vi "DriveModuleControl_TravTuneKsKv.vi"(8 "error in":errorcluster, 9 "Actual State":T1={"Speed"=0.0, "Angle"={"VALUE"=0.0, "COS"=1.0, "SIN"=0.0}} {"Angle"."SIN" format="%13.4f"; "Angle"."COS" format="%13.4f"; "Angle"."VALUE" format="%13.4f"}, 10 "Desired State":T1={"Speed"=0.0, "Angle"={"VALUE"=0.0, "COS"=1.0, "SIN"=0.0}} {"Angle"."SIN" format="%13.4f"; "Angle"."COS" format="%13.4f"; "Angle"."VALUE" format="%13.4f"}, 11 "ModualNamePrefix":i32) -> (0 "error out":errorcluster)   [LabVIEW 2023]
uses:
  <vilib>/Rock Robotics/WPI/ThirdParty/JAS_Junk/TrajLib/TypeDef/SWERVE_DRIVE_MODULE_STATE.ctl
  <vilib>/Rock Robotics/WPI/ThirdParty/JAS_Junk/TrajLib/TypeDef/ROTATION2D.ctl
  <vilib>/Rock Robotics/WPI/ThirdParty/JAS_Junk/TrajLib/LinearFilter_MovingAvg_Execute.vi
  <vilib>/Rock Robotics/WPI/ThirdParty/JAS_Junk/TrajLib/Rotation2d_Minus.vi
  <vilib>/Rock Robotics/WPI/ThirdParty/JAS_Junk/TrajLib/Rotation2d_GetRadians.vi
  <vilib>/Rock Robotics/WPI/ThirdParty/JAS_Junk/TrajLib/SwerveModuleState_New.vi
  <vilib>/Rock Robotics/WPI/ThirdParty/JAS_Junk/TrajLib/Rotation2d_RotateBy.vi
  <vilib>/Rock Robotics/WPI/ThirdParty/JAS_Junk/TrajLib/Rotation2d_CreateAngle.vi
  <vilib>/Rock Robotics/WPI/ThirdParty/JAS_Junk/TrajLib/SimpleMotorFF_Calculate.vi
  <vilib>/Rock Robotics/WPI/ThirdParty/JAS_Junk/TrajLib/LinearFilter_ResetToValue.vi
  <vilib>/Rock Robotics/WPI/ThirdParty/JAS_Junk/TrajLib/LinearFilter_Calculate.vi
  <vilib>/Rock Robotics/WPI/ThirdParty/JAS_Junk/TrajLib/PIDController_AtSetpoint.vi
  <vilib>/Rock Robotics/WPI/ThirdParty/JAS_Junk/TrajLib/PIDController_SetPIDF.vi
  <vilib>/Rock Robotics/WPI/ThirdParty/JAS_Junk/TrajLib/PIDController_SetDerivativeFilter.vi
  <vilib>/Rock Robotics/WPI/ThirdParty/JAS_Junk/TrajLib/PIDController_SetIntegratorRange.vi
  <vilib>/Rock Robotics/WPI/ThirdParty/JAS_Junk/TrajLib/PIDController_SetTolerancePandV.vi
  <vilib>/Rock Robotics/WPI/ThirdParty/JAS_Junk/TrajLib/PIDController_DisableContinousInput.vi
  <vilib>/Rock Robotics/WPI/ThirdParty/JAS_Junk/TrajLib/PIDController_EnableContinousInput.vi
  <vilib>/Rock Robotics/WPI/ThirdParty/JAS_Junk/TrajLib/PIDController_Reset.vi
  <vilib>/Rock Robotics/WPI/ThirdParty/JAS_Junk/TrajLib/PIDController_New.vi
  <vilib>/Rock Robotics/WPI/ThirdParty/JAS_Junk/TrajLib/PIDController_SetOutputLimits.vi
  <vilib>/Rock Robotics/WPI/ThirdParty/JAS_Junk/TrajLib/VI/PIDController_SetIntegratorZone.vi
  <vilib>/Rock Robotics/WPI/ThirdParty/JAS_Junk/TrajLib/Rotation2d_UnaryMinus.vi
  <vilib>/Rock Robotics/WPI/ThirdParty/JAS_Junk/TrajLib/Rotation2d_CreateXY.vi
  <vilib>/Rock Robotics/WPI/ThirdParty/JAS_Junk/TrajLib/PIDController_NewPeriod.vi
  <vilib>/Rock Robotics/WPI/ThirdParty/JAS_Junk/TrajLib/Util_CalcDist.vi
  <vilib>/Rock Robotics/SystemInterfaces/NetworkCommunication/NetComm_UsageReport_report.vi
  <vilib>/Rock Robotics/WPI/ThirdParty/Phoenix6/Phoenix6_Device_RefNumRegistryGet.vi
  <vilib>/Rock Robotics/WPI/MotorControl/WPI_MotorControlRefNum Registry Get.vi
  <vilib>/Rock Robotics/Network Tables/NT Write Number.vi
  DriveGlobal.vi
  <vilib>/Rock Robotics/WPI/ThirdParty/JAS_Junk/TrajLib/Globals/Util_LibraryGlobals.vi
  <vilib>/Rock Robotics/WPI/ThirdParty/JAS_Junk/TrajLib/PIDController_AdvCalculate_FF_Sp_Pv.vi
  <vilib>/Rock Robotics/WPI/ThirdParty/JAS_Junk/TrajLib/LinearFilter_MovingAverage.vi
  <vilib>/Utility/semaphor.llb/Obtain Semaphore Reference.vi
  <vilib>/Rock Robotics/WPI/ThirdParty/JAS_Junk/TrajLib/Timer_Reset.vi
  DriveTuningGlobals.vi
  <vilib>/Rock Robotics/WPI/ThirdParty/JAS_Junk/TrajLib/Trajectory_Library.lvlib
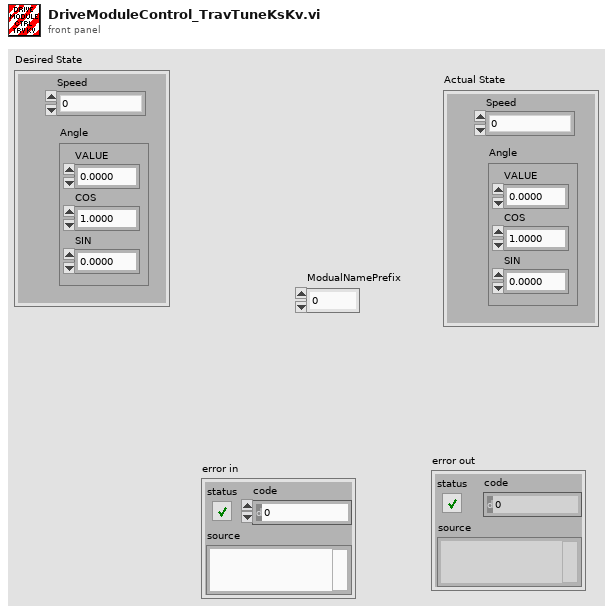
[diagram p1: front panel]
types:
  T1 = typedef "Trajectory_Library.lvlib/SWERVE_DRIVE_MODULE_STATE.ctl" = cluster{"Speed":dbl, "Angle":T2}
  T2 = typedef "Trajectory_Library.lvlib/ROTATION2D.ctl" = cluster{"VALUE":dbl, "COS":dbl, "SIN":dbl}
  T3 = typedef "WPI_MotorControlDeviceRef.ctl" = cluster{"DeviceStatus":errorcluster, "Type":T4, "PWM":cluster{"PWM Channel":T5, "DeadBand":T6}, "CAN":cluster{"Device Number":u8, "SetOutput VI Ref":variant, "GetOutput VI Ref":variant, "Enable VI Ref":variant, "Disable VI Ref":variant, "Data":variant}, "Invert":bool, "DIO PWM":cluster{"PWM \"Enable\" Channel":T5, "DIOChannel":T7, "PWM Rate":dbl}}
  T4 = typedef "WPI_MotorControlType.ctl" = enum16{"PWM", "CAN", "DIO PWM"}
  T5 = typedef "FPGA_DIOPWMChannel.ctl" = enum8{"PWM 0", "PWM 1", "PWM 2", "PWM 3", "PWM 4", "PWM 5", "PWM 6", "PWM 7", "PWM 8", "PWM 9", "PWM MXP 0", "PWM MXP 1", "PWM MXP 2", "PWM MXP 3", "PWM MXP 4", "PWM MXP 5", "PWM MXP 6", "PWM MXP 7", "PWM MXP 8", "PWM MXP 9", "Invalid"}
  T6 = typedef "WPI_PWMDeadband.ctl" = cluster{"Name":string, "maxPositivePwm":i32, "minPositivePwm":i32, "centerPwm":i32, "maxNegativePwm":i32, "minNegativePwm":i32, "angularRange":u16}
  T7 = typedef "FPGA_DIOChannel.ctl" = enum8{"DIO 0", "DIO 1", "DIO 2", "DIO 3", "DIO 4", "DIO 5", "DIO 6", "DIO 7", "DIO 8", "DIO 9", "DIO MXP 0", "DIO MXP 1", "DIO MXP 2", "DIO MXP 3", "DIO MXP 4", "DIO MXP 5", "DIO MXP 6", "DIO MXP 7", "DIO MXP 8", "DIO MXP 9", "DIO MXP 10", "DIO MXP 11", "DIO MXP 12", "DIO MXP 13", "DIO MXP 14", "DIO MXP 15", "SPI Port CS1", "SPI Port CS2", "SPI Port CS3", "SPI Port MISO", "SPI Port MOSI", "Invalid"}
  T8 = typedef "Trajectory_Library.lvlib/TIMER.ctl" = cluster{"StartTime":dbl, "Accumulated TIme":dbl, "Running":bool, "semaphore":T9}
  T9 = typedef "Semaphore RefNum" = refnum<k1>
  T10 = typedef "Trajectory_Library.lvlib/SIMPLE_MOTOR_FF.ctl" = cluster{"Ks":dbl, "Kv":dbl, "Ka":dbl, "KnInv":dbl}
  T11 = typedef "Trajectory_Library.lvlib/PID_ADV_LIMITS.ctl" = cluster{"MaxInput":dbl, "MinInput":dbl, "Continuous":bool, "MaxOutput":dbl, "MinOutput":dbl}
  T12 = typedef "Trajectory_Library.lvlib/PID_ADV_TUNING.ctl" = cluster{"Kf":dbl, "Kp":dbl, "Ki":dbl, "Kd":dbl, "MaximumIntegral":dbl, "MinimumIntegral":dbl, "Filter Derivative":bool, "IntegralZone":dbl}
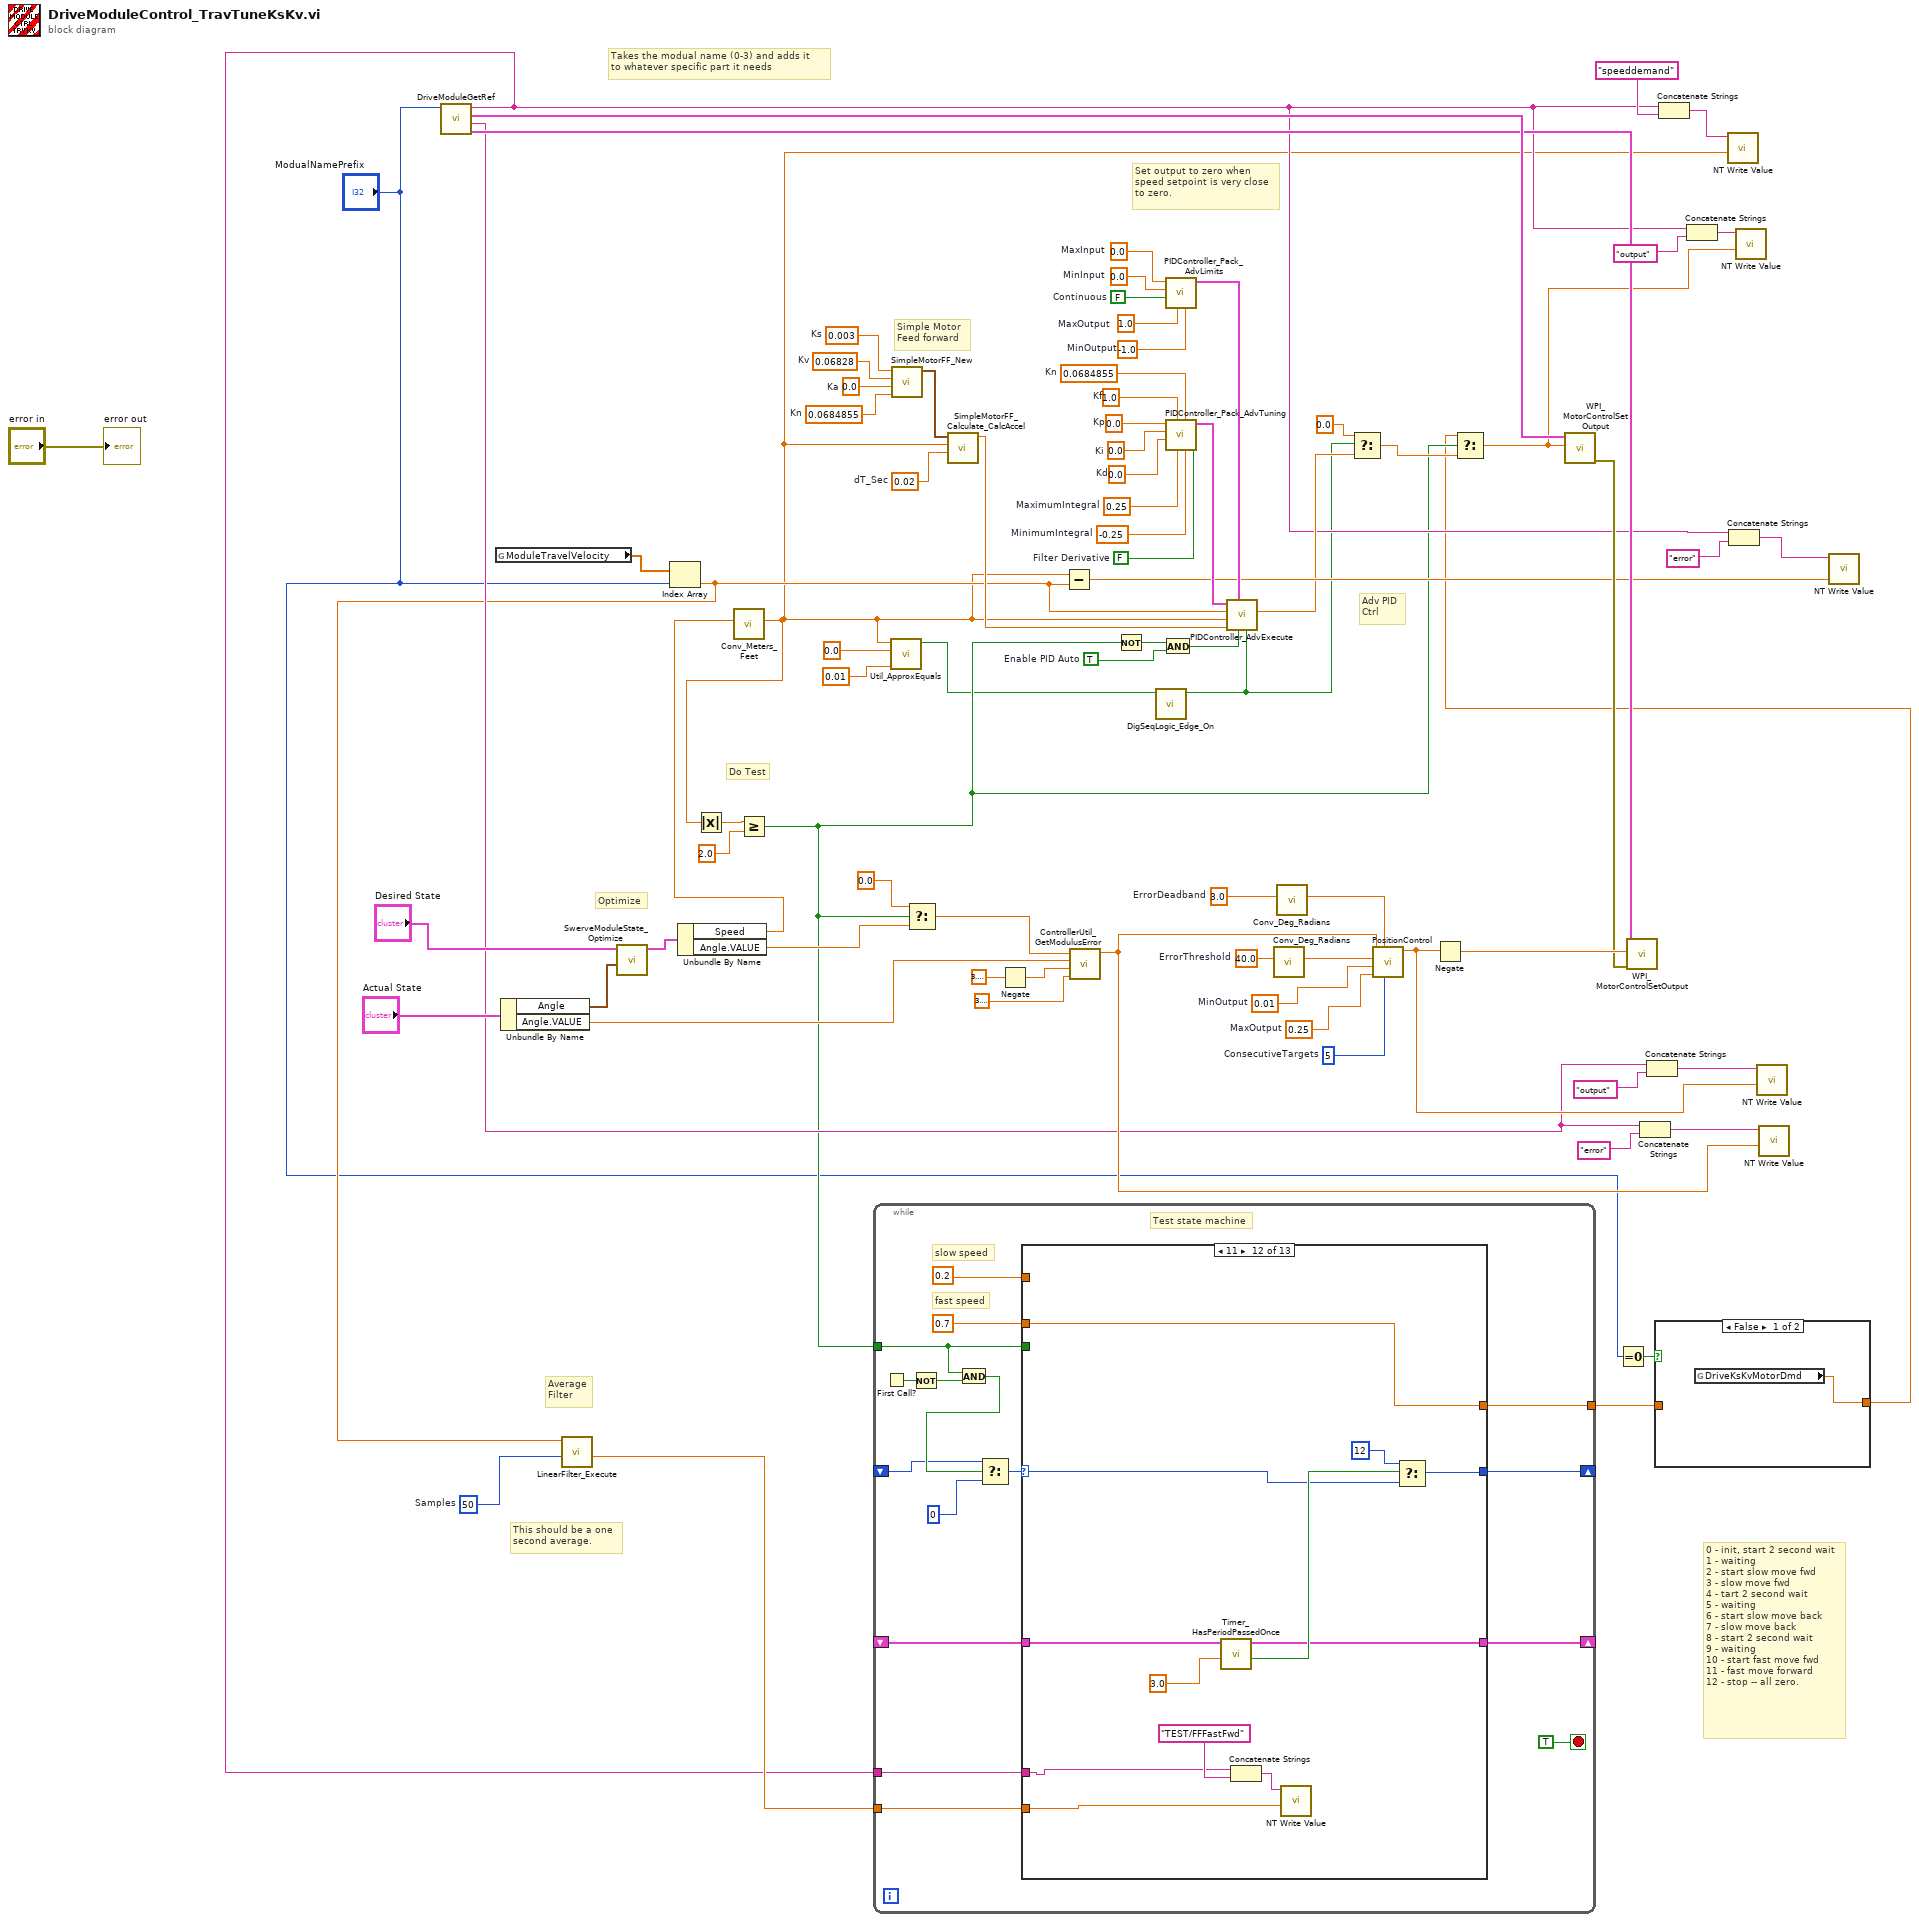
[diagram p0: block diagram]
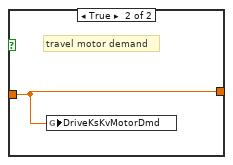
[diagram p2: hidden frame]
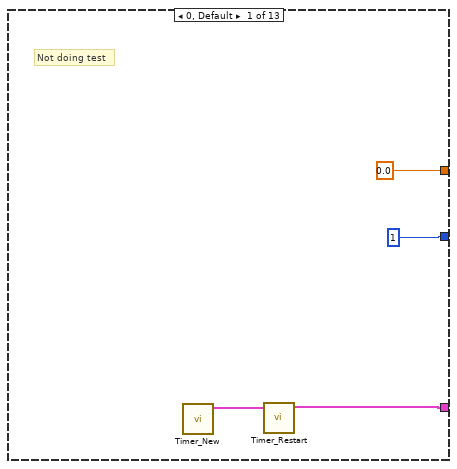
[diagram p3: hidden frame]
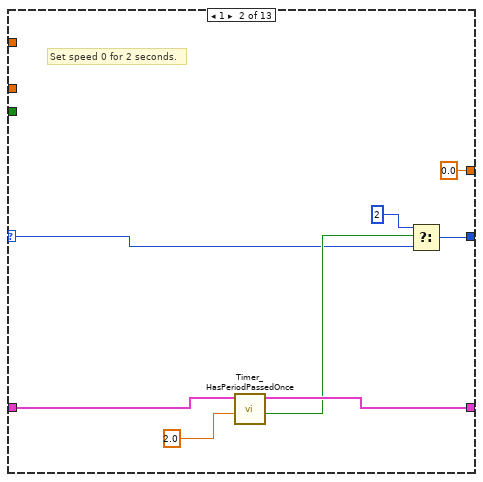
[diagram p4: hidden frame]
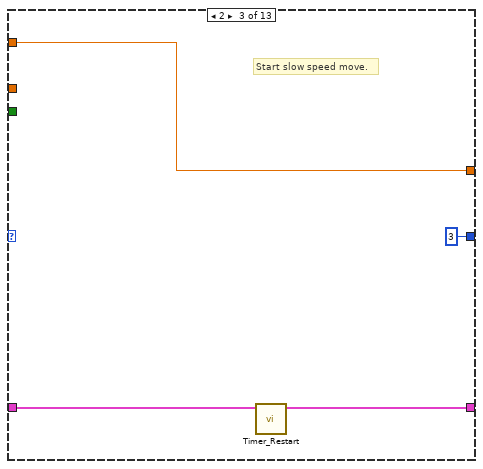
[diagram p5: hidden frame]
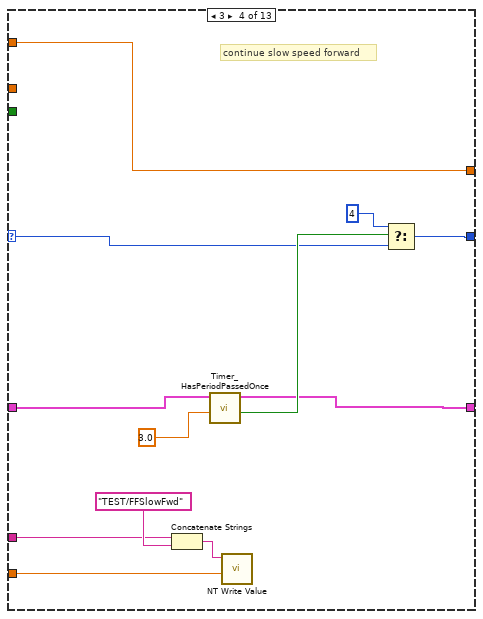
[diagram p6: hidden frame]
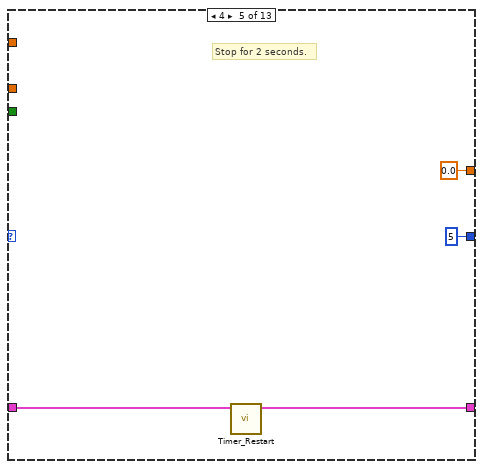
[diagram p7: hidden frame]
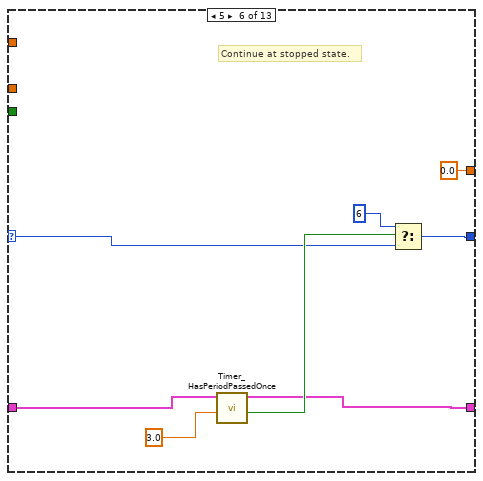
[diagram p8: hidden frame]
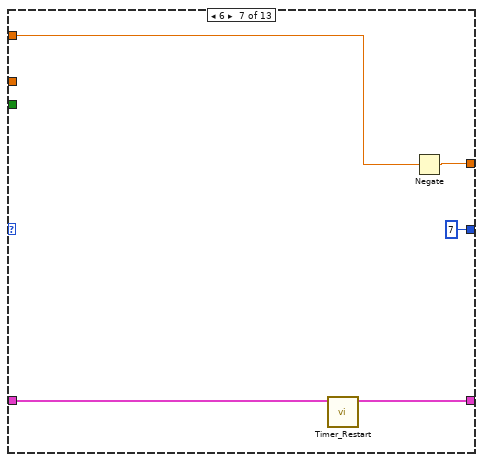
[diagram p9: hidden frame]
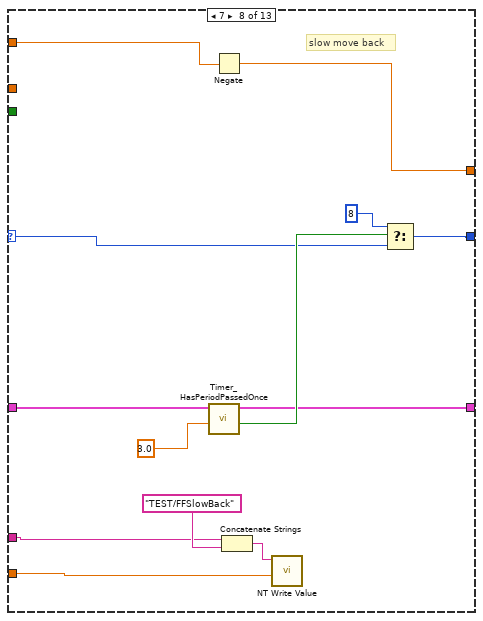
[diagram p10: hidden frame]
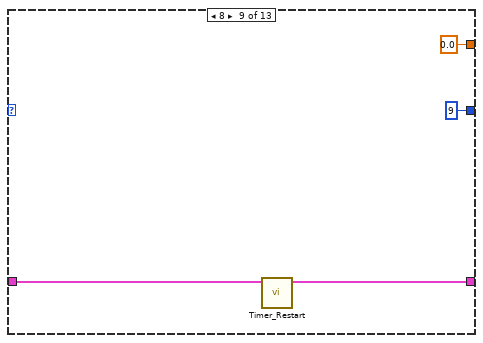
[diagram p11: hidden frame]
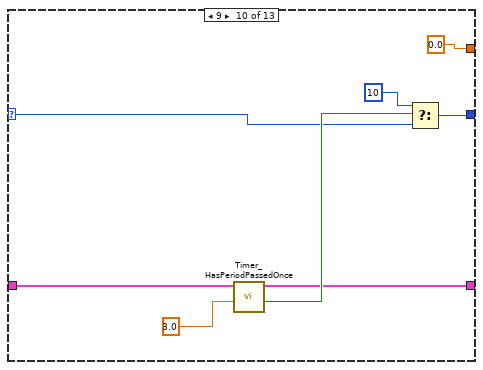
[diagram p12: hidden frame]
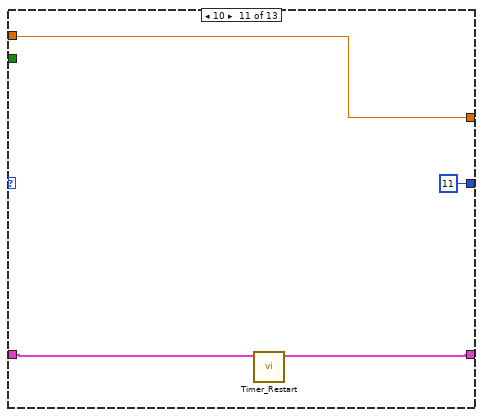
[diagram p13: hidden frame]
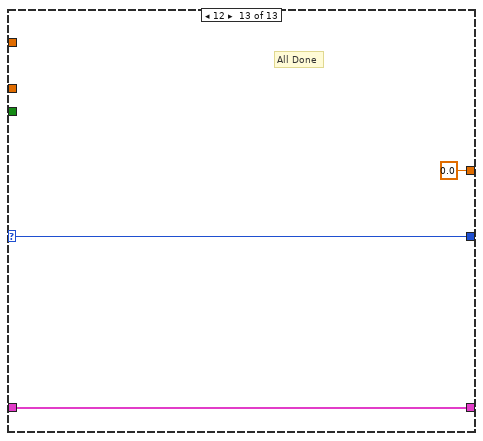
[diagram p14: hidden frame]
diagram:
  w8 = 50  # Samples
  w23 = TRUE  # Enable PID Auto
  w32 = 0.0684855  # Kn
  w48 = 0.0  # Kp
  w47 = 0.0  # Ki
  w46 = 0.0  # Kd
  w45 = 1.0  # Kf
  w44 = 0.25  # MaximumIntegral
  w43 = -0.25  # MinimumIntegral
  w42 = FALSE  # Filter Derivative
  w40 = 0.0  # MinInput
  w39 = FALSE  # Continuous
  w38 = 1.0  # MaxOutput
  w41 = -1.0  # MinOutput
  w37 = 0.0  # MaxInput
  w57 = 0.0684855  # Kn
  w56 = 0.02  # dT_Sec
  w54 = 0.003  # Ks
  w53 = 0.06828  # Kv
  w52 = 0.0  # Ka
  w67 = 5  # ConsecutiveTargets
  w64 = 0.25  # MaxOutput
  w68 = 0.01  # MinOutput
  w61 = 40.0  # ErrorThreshold
  w63 = 3.0  # ErrorDeadband
  # "This should be a one\nsecond average."
  # "Average\nFilter"
  # "0 - init, start 2 second wait\n1 - waiting\n2 - start slow move fwd\n3 - slow move fwd\n4 - tart 2 second wait\n5 - waiting\n6 - start slow move back\n7 - slow move back\n8 - start 2 second wait\n9 - waiting\n10 - start fast move fwd\n11 - fast move forward\n12 - stop -- all zero."
  # "Do Test"
  # "Optimize"
  # "Set output to zero when\nspeed setpoint is very close\nto zero."
  # "Adv PID\nCtrl"
  # "Simple Motor\nFeed forward"
  # "Takes the modual name (0-3) and adds it \nto whatever specific part it needs"
  n1 = call "DriveModuleGetRef.vi"("ModualNamePrefix"="ModualNamePrefix") -> ("SpinMot"=w49:T3, "SpinStr"=w28:string, "TravMot"=w50:T3, "TravStr"=w10:string)  [unwired: 5 in, 2 out]
  n2 = global read "DriveGlobal.vi" "ModuleTravelVelocity"() -> (w33:dbl[])
  n3 = Unbundle By Name("Actual State") -> ("Angle"=w74:T2, "Angle.VALUE"=w71:dbl)
  n4 = call <vilib>:"SwerveModuleState_Optimize.vi"("CurrentAngle"=w74, "Desired State"="Desired State") -> ("out SWERVE_DRIVE_MODULE_STATE"=w72:T1)  [unwired: 9 in]
  n5 = Index Array(array=w33, index="ModualNamePrefix") -> (element=w12:dbl)
  n6 = call-poly <vilib>:"LinearFilter_Execute.vi"("Samples"=w8, "Input"=w12) -> ("Output"=w11:dbl)  [unwired: 9 in]
  n7 = Unbundle By Name(w72) -> ("Speed"=w20:dbl, "Angle.VALUE"=w17:dbl)
  n8 = call <vilib>:"Conv_Meters_Feet.vi"("Meters"=w20) -> ("Feet"=w3:dbl)  [unwired: 10 in]
  n9 = Absolute Value(x=w3) -> (abs(x)=w19:dbl)
  n10 = Greater Or Equal?(x=w19, y=2.0) -> (x >= y?=w9:bool)
  n11 = while {
    shift-right: [w99] -> _
    shift-left: _ -> [w91]
    shift-right: [w98] -> _
    shift-left: _ -> [w89]
    tunnel: w9 -> [w93]
    tunnel: [w90] -> w7
    tunnel: w11 -> [w86]
    tunnel: w10 -> [w85]
    stop <- TRUE stop-if-true
    # "fast speed"
    # "slow speed"
    # "Test state machine"
    n12 = First Call?() -> (First Call?: T/F=w95:bool)
    n13 = Not(x=w95) -> (.not. x?=w94:bool)
    n14 = And(x=w93, y=w94) -> (x .and. y?=w92:bool)
    n15 = Select(t=w91, s=w92, f=0 ("t")) -> (s? t:f=w97:i32)
    n16 = case shown="11" w97 {
      selector: w97 -> [_ w107 _ w124 _ w136 _ w152 _ w163 _ w179 w188]
      tunnel: [1 w106 3 ("t") w125 5 ("t") w137 7 ("t") w153 9 ("t") w167 11 ("t") w182 w188] -> w99
      tunnel: [w103 w110 w114 w122 w130 w134 w145 w150 w160 w165 w171 w180 w187] -> w98
      tunnel: w93 -> [_ _ _ _ _ _ _ _ _ _ _ _ _]
      tunnel: [0.0 0.0 w113 w121 0.0 0.0 w142 w157 0.0 0.0 w174 w186 0.0] -> w90
      tunnel: w89 -> [_ w111 w115 w123 w131 w135 w144 w151 w159 w166 w172 w181 w187]
      tunnel: 0.2 -> [_ _ w113 w121 _ _ w141 w158 _ _ _ _ _]
      tunnel: 0.7 -> [_ _ _ _ _ _ _ _ _ _ w174 w186 _]
      tunnel: w86 -> [_ _ _ w120 _ _ _ w146 _ _ _ w175 _]
      tunnel: w85 -> [_ _ _ w117 _ _ _ w147 _ _ _ w176 _]
      frame 0, Default {
        # "Not doing test"
        n17 = call <vilib>:"Timer_New.vi"() -> ("TIMER"=w104:T8)  [unwired: 11 in]
        n18 = call <vilib>:"Timer_Restart.vi"("in Timer"=w104) -> ("out Timer"=w103:T8)  [unwired: 10 in]
      }
      frame 1 {
        # "Set speed 0 for 2 seconds."
        n19 = call <vilib>:"Timer_HasPeriodPassedOnce.vi"("Period"=2.0, "in Timer"=w111) -> ("Expired"=w108:bool, "out Timer"=w110:T8)  [unwired: 7 in, 1 out]
        n20 = Select(t=2, s=w108, f=w107) -> (s? t:f=w106:i32)
      }
      frame 2 {
        # "Start slow speed move."
        n21 = call <vilib>:"Timer_Restart.vi"("in Timer"=w115) -> ("out Timer"=w114:T8)  [unwired: 10 in]
      }
      frame 3 {
        # "continue slow speed forward"
        n22 = Concatenate Strings(w117, "TEST/FFSlowFwd" ("refnum name")) -> (w118:string)
        n23 = call <vilib>:"Timer_HasPeriodPassedOnce.vi"("Period"=3.0, "in Timer"=w123) -> ("Expired"=w127:bool, "out Timer"=w122:T8)  [unwired: 7 in, 1 out]
        n24 = call-poly <vilib>:"NT Write Value.vi"("value"=w120, "name"=w118) -> ()  [unwired: 9 in, 1 out]
        n25 = Select(t=4, s=w127, f=w124) -> (s? t:f=w125:i32)
      }
      frame 4 {
        # "Stop for 2 seconds."
        n26 = call <vilib>:"Timer_Restart.vi"("in Timer"=w131) -> ("out Timer"=w130:T8)  [unwired: 10 in]
      }
      frame 5 {
        # "Continue at stopped state."
        n27 = call <vilib>:"Timer_HasPeriodPassedOnce.vi"("Period"=3.0, "in Timer"=w135) -> ("Expired"=w139:bool, "out Timer"=w134:T8)  [unwired: 7 in, 1 out]
        n28 = Select(t=6, s=w139, f=w136) -> (s? t:f=w137:i32)
      }
      frame 6 {
        n29 = call <vilib>:"Timer_Restart.vi"("in Timer"=w144) -> ("out Timer"=w145:T8)  [unwired: 10 in]
        n30 = Negate(x=w141) -> (-x=w142:dbl)
      }
      frame 7 {
        # "slow move back"
        n31 = call <vilib>:"Timer_HasPeriodPassedOnce.vi"("Period"=3.0, "in Timer"=w151) -> ("Expired"=w155:bool, "out Timer"=w150:T8)  [unwired: 7 in, 1 out]
        n32 = Negate(x=w158) -> (-x=w157:dbl)
        n33 = Concatenate Strings(w147, "TEST/FFSlowBack" ("refnum name")) -> (w148:string)
        n34 = call-poly <vilib>:"NT Write Value.vi"("value"=w146, "name"=w148) -> ()  [unwired: 9 in, 1 out]
        n35 = Select(t=8, s=w155, f=w152) -> (s? t:f=w153:i32)
      }
      frame 8 {
        n36 = call <vilib>:"Timer_Restart.vi"("in Timer"=w159) -> ("out Timer"=w160:T8)  [unwired: 10 in]
      }
      frame 9 {
        n37 = call <vilib>:"Timer_HasPeriodPassedOnce.vi"("Period"=3.0, "in Timer"=w166) -> ("Expired"=w169:bool, "out Timer"=w165:T8)  [unwired: 7 in, 1 out]
        n38 = Select(t=10, s=w169, f=w163) -> (s? t:f=w167:i32)
      }
      frame 10 {
        n39 = call <vilib>:"Timer_Restart.vi"("in Timer"=w172) -> ("out Timer"=w171:T8)  [unwired: 10 in]
      }
      frame 11 {
        n40 = call <vilib>:"Timer_HasPeriodPassedOnce.vi"("Period"=3.0, "in Timer"=w181) -> ("Expired"=w184:bool, "out Timer"=w180:T8)  [unwired: 7 in, 1 out]
        n41 = Concatenate Strings(w176, "TEST/FFFastFwd" ("refnum name")) -> (w177:string)
        n42 = call-poly <vilib>:"NT Write Value.vi"("value"=w175, "name"=w177) -> ()  [unwired: 9 in, 1 out]
        n43 = Select(t=12, s=w184, f=w179) -> (s? t:f=w182:i32)
      }
      frame 12 {
        # "All Done"
      }
    }
  }
  n44 = call <vilib>:"Util_ApproxEquals.vi"("Tolerance"=0.01, "Value 2"=0.0, "Value 1"=w3) -> ("ApproxEquals"=w2:bool)  [unwired: 8 in]
  n45 = call <vilib>:"SimpleMotorFF_New.vi"("Kn"=w57, "Ka"=w52, "Kv"=w53, "Ks"=w54) -> ("SIMPLE_MOTOR_FF"=w55:T10)  [unwired: 7 in]
  n46 = Select(t=0.0, s=w9, f=w17) -> (s? t:f=w13:dbl)
  n47 = call <vilib>:"SimpleMotorFF_Calculate_CalcAccel.vi"("dT_Sec"=w56, "VelSp"=w3, "SIMPLE_MOTOR_FF"=w55) -> ("FeedForward"=w34:dbl)  [unwired: 8 in]
  n48 = Negate(x=3.141592653589793) -> (-x=w73:dbl)
  n49 = Subtract(x=w3, y=w12) -> (x-y=w29:dbl)
  n50 = call <vilib>:"ControllerUtil_GetModulusError.vi"("Maximum_Input"=3.141592653589793, "Minimum_Input"=w73, "Measurerment(PV)"=w71, "Reference(SP)"=w13) -> ("Error"=w65:dbl)  [unwired: 7 in]
  n51 = Not(x=w9) -> (.not. x?=w24:bool)
  n52 = call <vilib>:"DigSeqLogic_Edge_On.vi"("Input"=w2) -> ("On Edge"=w1:bool)  [unwired: 10 in]
  n53 = And(x=w24, y=w23) -> (x .and. y?=w25:bool)
  n54 = call <vilib>:"PIDController_Pack_AdvLimits.vi"("MinOutput"=w41, "MaxOutput"=w38, "Continuous"=w39, "MinInput"=w40, "MaxInput"=w37) -> ("Adv PID Limits"=w35:T11)  [unwired: 6 in]
  n55 = call <vilib>:"PIDController_Pack_AdvTuning.vi"("Filter Derivative"=w42, "MinimumIntegral"=w43, "Kn"=w32, "MaximumIntegral"=w44, "Kf"=w45, "Kd"=w46, "Ki"=w47, "Kp"=w48) -> ("Adv PID Tuning"=w36:T12)  [unwired: 3 in]
  n56 = call <vilib>:"PIDController_AdvExecute.vi"("Reset"=w1, "Auto"=w25, "Adv PID Limits"=w35, "FF-FeedForward"=w34, "SP-SetPoint"=w3, "PV-Measurement"=w12, "Adv PID Tuning"=w36) -> ("CO-ControlOutput"=w22:dbl)  [unwired: 2 in, 2 out]
  n57 = call <vilib>:"Conv_Deg_Radians.vi"("Degress"=w61) -> ("Radians"=w60:dbl)  [unwired: 10 in]
  n58 = call <vilib>:"Conv_Deg_Radians.vi"("Degress"=w63) -> ("Radians"=w62:dbl)  [unwired: 10 in]
  n59 = Select(t=0.0, s=w1, f=w22) -> (s? t:f=w14:dbl)
  n60 = call "PositionControl.vi"("ConsecutiveTargets"=w67, "ErrorDeadband"=w62, "MaxOutput"=w64, "MinOutput"=w68, "ErrorThreshold"=w60, "Error"=w65) -> ("OutputValue"=w59:dbl)  [unwired: 3 in, 2 out]
  n61 = Negate(x=w59) -> (-x=w58:dbl)
  n62 = Equal To 0?(x="ModualNamePrefix") -> (x = 0?=w6:bool)
  n63 = Concatenate Strings(w28, "error" ("refnum name")) -> (w78:string)
  n64 = Concatenate Strings(w28, "output" ("refnum name")) -> (w66:string)
  n65 = case shown="False" w6 {
    tunnel: w7 -> [_ w191]
    tunnel: [w190 w191] -> w4
    frame False {
      n66 = global read "DriveTuningGlobals.vi" "DriveKsKvMotorDmd"() -> (w190:dbl)
    }
    frame True {
      # "travel motor demand"
      n67 = global write "DriveTuningGlobals.vi" "DriveKsKvMotorDmd"(w191) -> ()
    }
  }
  n68 = Select(t=w4, s=w9, f=w14) -> (s? t:f=w15:dbl)
  n69 = call <vilib>:"WPI_MotorControlSetOutput.vi"("Output"=w15, "MotorControlDevRef"=w50) -> ("error out"=w51:errorcluster)  [unwired: 7 in, 2 out]
  n70 = call <vilib>:"WPI_MotorControlSetOutput.vi"("error in (no error)"=w51, "Output"=w58, "MotorControlDevRef"=w49) -> ()  [unwired: 6 in, 3 out]
  n71 = Concatenate Strings(w10, "speeddemand" ("refnum name")) -> (w82:string)
  n72 = Concatenate Strings(w10, "output" ("refnum name")) -> (w80:string)
  n73 = call-poly <vilib>:"NT Write Value.vi"("value"=w3, "name"=w82) -> ()  [unwired: 9 in, 1 out]
  n74 = Concatenate Strings(w10, "error" ("refnum name")) -> (w30:string)
  n75 = call-poly <vilib>:"NT Write Value.vi"("value"=w15, "name"=w80) -> ()  [unwired: 9 in, 1 out]
  n76 = call-poly <vilib>:"NT Write Value.vi"("value"=w59, "name"=w66) -> ()  [unwired: 9 in, 1 out]
  n77 = call-poly <vilib>:"NT Write Value.vi"("value"=w65, "name"=w78) -> ()  [unwired: 9 in, 1 out]
  n78 = call-poly <vilib>:"NT Write Value.vi"("value"=w29, "name"=w30) -> ()  [unwired: 9 in, 1 out]
  "error out" <- "error in"
